vi "SaveSettings.vi"(11 "Settings":T1 {"Max reports to save" min=1}) -> ()   [LabVIEW 2020, in "DependencyViewer.lvlib"]
uses:
  DependencyViewer.lvlib
  Settings.ctl
  DependencyConfiguration.ctl
  FilterOptions.ctl
  Viewer.ctl
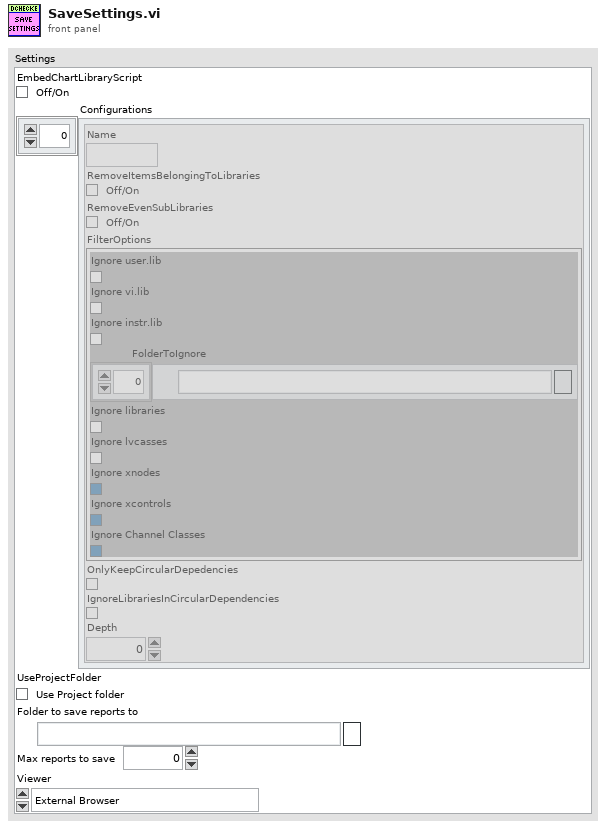
[diagram p1: front panel]
types:
  T1 = typedef "DependencyViewer.lvlib/Settings.ctl" = cluster{"EmbedChartLibraryScript":bool, "Configurations":T2[], "UseProjectFolder":bool, "Folder to save reports to":path, "Max reports to save":u8, "Viewer":T4}
  T2 = typedef "DependencyViewer.lvlib/DependencyConfiguration.ctl" = cluster{"Name":string, "RemoveItemsBelongingToLibraries":bool, "RemoveEvenSubLibraries":bool, "FilterOptions":T3, "OnlyKeepCircularDepedencies":bool, "IgnoreLibrariesInCircularDependencies":bool, "Depth":i32}
  T3 = typedef "DependencyViewer.lvlib/FilterOptions.ctl" = cluster{"Ignore user.lib":bool, "Ignore vi.lib":bool, "Ignore instr.lib":bool, "FolderToIgnore":path[], "Ignore libraries":bool, "Ignore lvcasses":bool, "Ignore xnodes":bool, "Ignore xcontrols":bool, "Ignore Channel Classes":bool}
  T4 = typedef "DependencyViewer.lvlib/Viewer.ctl" = enum16{"External Browser", "Integrated WebView2 Browser"}
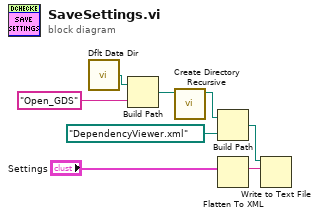
[diagram p0: block diagram]
diagram:
  n1 = call <vilib>:"Dflt Data Dir.vi"() -> ("App:Default Data Directory"=w6:path)
  n2 = Build Path(base path=w6, name or relative path="Open_GDS") -> (appended path=w7:path)
  n3 = call <vilib>:"Create Directory Recursive.vi"("directory"=w7) -> ("directory copy"=w2:path)  [unwired: 4 in, 2 out]
  n4 = Build Path(base path=w2, name or relative path=path "DependencyViewer.xml") -> (appended path=w3:path)
  n5 = Flatten To XML(6:"Settings") -> (2:w8:string)
  n6 = Write to Text File(file (use dialog)=w3, text=w8) -> ()  [unwired: 2 in, 3 out]
